vi "(TestVI)DW7912 Memory Read.vi"() -> ()   [LabVIEW 2020]
uses:
  SubVIs/Serial/Controls/(Ctrl)Serial_FGV Function.ctl
  <vilib>/Instr/_visa.llb/VISA Find Search Mode.ctl
  ad51c9fb-ed1b-493e-b3a3-f21aa68cfd60.vi
  SubVIs/I2C/Instance VIs/(SubVI)I2C_8Bit-8Bit_Write_Sequential.vi
  SubVIs/I2C/Instance VIs/(SubVI)I2C_8Bit-8Bit_Read_Sequential.vi
panel:
  out "Read Data 4":u8[](array[numeric])
  out "Read Data 3":u8[](array[numeric])
  out "Read Data 2":u8[](array[numeric])
  out "Read Data":u8[](array[numeric])
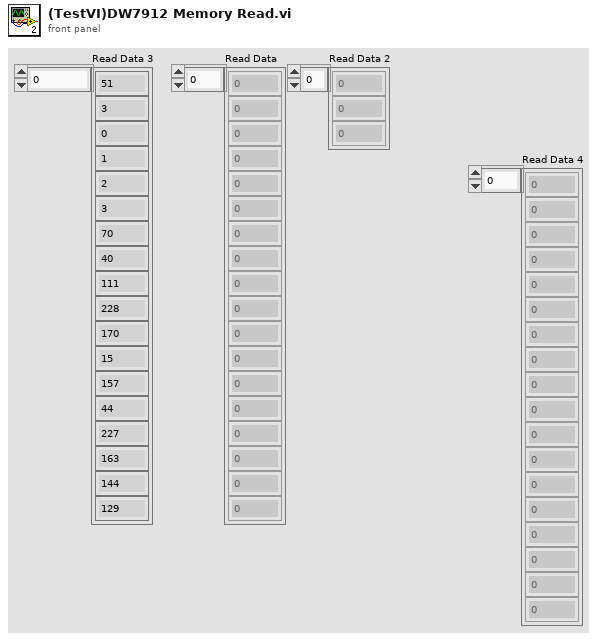
[diagram p1: front panel]
types:
  T1 = typedef "VISA Find Search Mode.ctl" = u32
  T2 = typedef "(Ctrl)Serial_FGV Function.ctl" = enum16{"Initialize", "Read", "Read All", "Write", "Flush Buffer", "Get Ref.", "Close"}
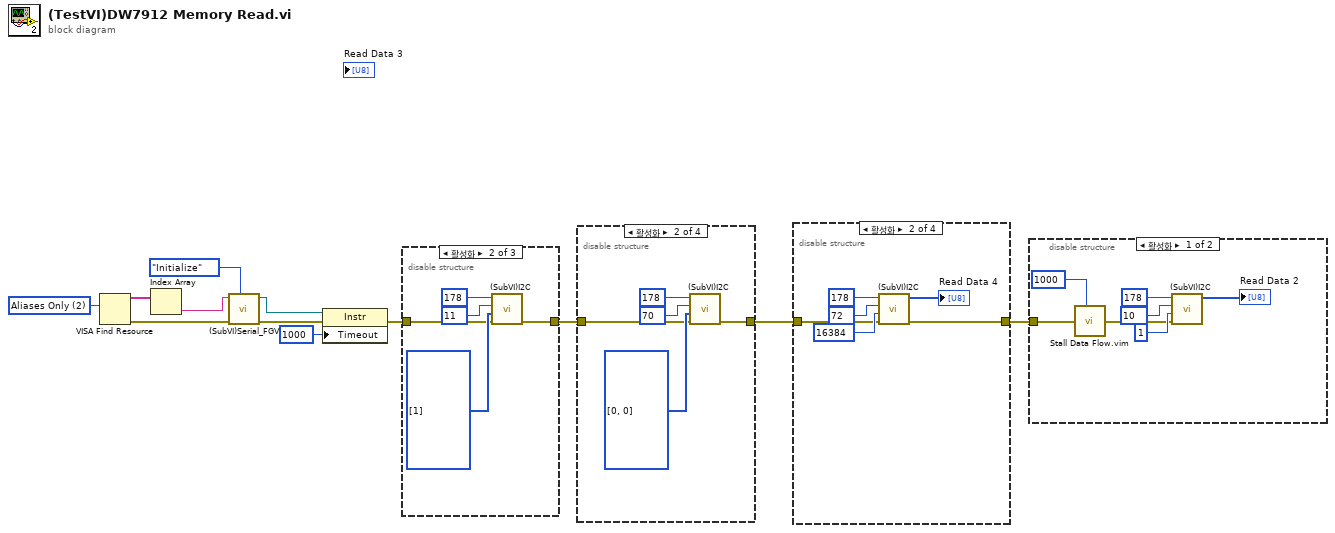
[diagram p0: block diagram]
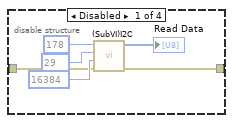
[diagram p2: hidden frame]
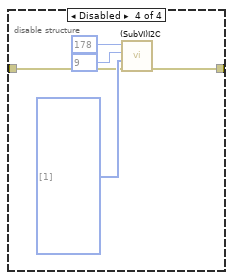
[diagram p4: hidden frame]
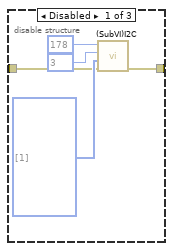
[diagram p6: hidden frame]
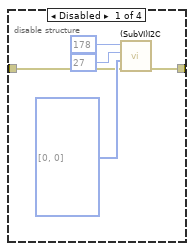
[diagram p8: hidden frame]
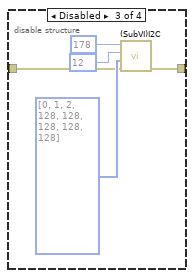
[diagram p9: hidden frame]
diagram:
  w11 = T1 2 items=["Canonical Names Only"=0, "Aliases Only"=2, "Include Matching Aliases"=3, "Include All Aliases"=4] ("Search Mode")
  n1 = VISA Find Resource(10:w11) -> (0:w10:errorcluster, 3:w9:string[])  [unwired: 2 in, 1 out]
  n2 = Index Array(array=w9) -> (element=w8:string)  [unwired: 1 in]
  n3 = call "(SubVI)Serial_FGV.vi"("Function"=(Ctrl)Serial_FGV_Function."Initialize", "error in (no error)"=w10, "VISA resource name"=w8) -> ("error out"=w7:errorcluster, "VISA resource name out"=w6:refnum<visa-resource-name>)  [unwired: 6 in, 1 out]
  n4 = property class="Instr"(reference=w6, error in=w7, "Timeout"=u32 1000 ("General Settings:Timeout Value")) -> (error out=w3:errorcluster)  [unwired: 1 out]
  n5 = disable-structure shown="활성화" {
    disable-tunnel: w3 -> [w14 w19 w23]
    disable-tunnel: [w13 w18 w23] -> w2
    frame Disabled {
      n6 = call-poly "(SubVI)I2C.vi"("error in (no error)"=w14, "Data to Write"=u8[] [1] ("Size to Read"), "Start Address"=u8 3, "ID"=u8 178) -> ("error out"=w13:errorcluster)  [unwired: 6 in, 1 out]
    }
    frame Enabled {
      n7 = call-poly "(SubVI)I2C.vi"("error in (no error)"=w19, "Data to Write"=u8[] [1] ("Size to Read"), "Start Address"=u8 11, "ID"=u8 178) -> ("error out"=w18:errorcluster)  [unwired: 6 in, 1 out]
    }
    frame Disabled {
    }
  }
  n8 = disable-structure shown="활성화" {
    disable-tunnel: [w25 w30 w35 w39] -> w4
    disable-tunnel: w2 -> [w24 w29 w34 w39]
    frame Disabled {
      n9 = call-poly "(SubVI)I2C.vi"("error in (no error)"=w24, "Data to Write"=u8[] [0, 0] ("Size to Read"), "Start Address"=u8 27, "ID"=u8 178) -> ("error out"=w25:errorcluster)  [unwired: 6 in, 1 out]
    }
    frame Enabled {
      n10 = call-poly "(SubVI)I2C.vi"("error in (no error)"=w29, "Data to Write"=u8[] [0, 0] ("Size to Read"), "Start Address"=u8 70, "ID"=u8 178) -> ("error out"=w30:errorcluster)  [unwired: 6 in, 1 out]
    }
    frame Disabled {
      n11 = call-poly "(SubVI)I2C.vi"("error in (no error)"=w34, "Data to Write"=u8[] [0, 1, 2, 128, 128, 128, 128, 128] ("Size to Read"), "Start Address"=u8 12, "ID"=u8 178) -> ("error out"=w35:errorcluster)  [unwired: 6 in, 1 out]
    }
    frame Disabled {
    }
  }
  n12 = disable-structure shown="활성화" {
    disable-tunnel: w4 -> [w42 w48 w52 w54]
    disable-tunnel: [w41 w47 w52 w53] -> w1
    frame Disabled {
      n13 = call-poly "(SubVI)I2C.vi"("error in (no error)"=w42, "Size to Read"=u16 16384, "Start Address"=u8 29, "ID"=u8 178) -> ("error out"=w41:errorcluster, "Read Data"=→"Read Data":u8[])  [unwired: 5 in, 1 out]
    }
    frame Enabled {
      n14 = call-poly "(SubVI)I2C.vi"("error in (no error)"=w48, "Size to Read"=u16 16384, "Start Address"=u8 72, "ID"=u8 178) -> ("error out"=w47:errorcluster, "Read Data"=→"Read Data 4":u8[])  [unwired: 5 in, 1 out]
    }
    frame Disabled {
    }
    frame Disabled {
      n15 = call-poly "(SubVI)I2C.vi"("error in (no error)"=w54, "Data to Write"=u8[] [1] ("Size to Read"), "Start Address"=u8 9, "ID"=u8 178) -> ("error out"=w53:errorcluster)  [unwired: 6 in, 1 out]
    }
  }
  n16 = disable-structure shown="활성화" {
    disable-tunnel: w1 -> [w61 _]
    frame Enabled {
      n17 = call "Stall Data Flow.vim"("value in"=w61, "milliseconds to wait"=u32 1000) -> ("value out"=w59:errorcluster)  [unwired: 1 out]
      n18 = call-poly "(SubVI)I2C.vi"("error in (no error)"=w59, "Size to Read"=u16 1, "Start Address"=u8 10, "ID"=u8 178) -> ("Read Data"=→"Read Data 2":u8[])  [unwired: 5 in, 2 out]
    }
    frame Disabled {
    }
  }
